vi "CallFacialClassificationFunction_IMA_DEPRECATEDQ.vi"(8 "error in (no error)":errorcluster, 9 "Function or Method Name":string="find_faces", 10 "image":T1, 11 "reference in":refnum<class "ImageFacialDetection.lvclass">) -> (0 "error out":errorcluster, 2 "image with faces":T1, 3 "reference out":refnum<class "ImageFacialDetection.lvclass">)   [LabVIEW 2017]
doc: "uses the image classification in python with openCV to detect faces in an image using Haar Cascades"
uses:
  ImageFacialDetection.lvclass
  <vilib>/Enthought/Python Integration Toolkit/Python Integration Toolkit.lvlib
  <vilib>/Enthought/Python Integration Toolkit/api/Unpack As Variant.vi
  <vilib>/vision/Image Controls.llb/IMAQ Image.ctl
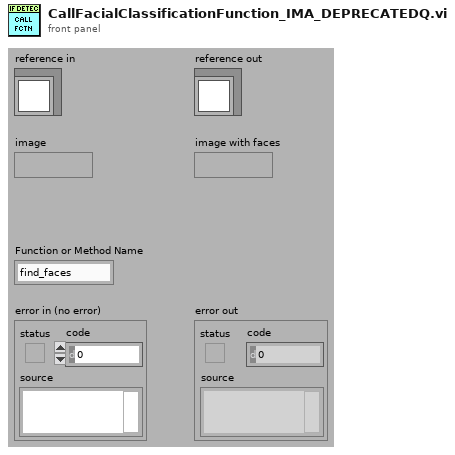
[diagram p1: front panel]
types:
  T1 = typedef "IMAQ Image.ctl" = refnum<image>
  T2 = typedef "Python Integration Toolkit.lvlib/Session ID.ctl" = u64
  T3 = typedef "Python Integration Toolkit.lvlib/Python Objects.ctl" = variant
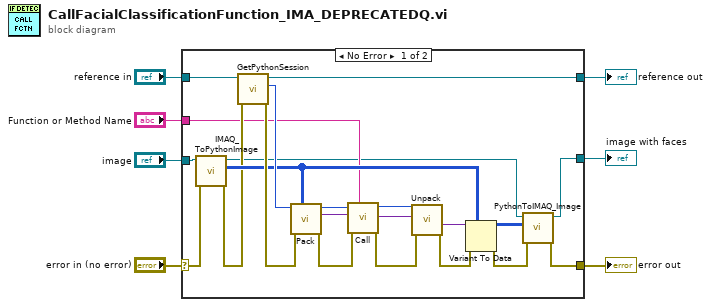
[diagram p0: block diagram]
diagram:
  n1 = case shown="No Error" "error in (no error)" {
    selector: "error in (no error)" -> [w18 w31]
    tunnel: [w11 w31] -> w6
    tunnel: [w28 w30] -> w4
    tunnel: "reference in" -> [w29 w30]
    tunnel: "image" -> [w27 _]
    tunnel: [w13 _] -> w2
    tunnel: "Function or Method Name" -> [w9 _]
    frame No Error {
      n2 = call "IMAQ_ToPythonImage.vi"("error in (no error)"=w18, "IMAQ Image in"=w27) -> ("error out"=w17:errorcluster, "Python Image Data"=w19:u8[][][], "IMAQ Image dup"=w8:T1)  [unwired: 7 in]
      n3 = call "GetPythonSession.vi"("error in (no error)"=w17, "reference in"=w29) -> ("error out"=w25:errorcluster, "Python Session ID"=w26:T2, "reference out"=w28:refnum<class "ImageFacialDetection.lvclass">)  [unwired: 7 in]
      n4 = call <vilib>:"Pack.vi"("Argument"=w19, "error in (no error)"=w25, "Session ID"=w26) -> ("error out"=w22:errorcluster, "Python Object References Out"=w23:T3, "Session ID out"=w24:T2)  [unwired: 6 in]
      n5 = call <vilib>:"Call.vi"("Function or Method Name"=w9, "error in (no error)"=w22, "Python Object References In"=w23, "Session ID"=w24) -> ("error out"=w15:errorcluster, "Python Object References Out"=w20:T3, "Session ID out"=w21:T2)  [unwired: 5 in]
      n6 = call-poly <vilib>:"Unpack.vi"("error in (no error)"=w15, "Python Object References In"=w20, "Session ID"=w21) -> ("error out"=w14:errorcluster, "Value"=w10:variant)  [unwired: 5 in, 2 out]
      n7 = Variant To Data(error in=w14, type=w19, Variant=w10) -> (data=w16:u8[][][], error out=w12:errorcluster)
      n8 = call "PythonToIMAQ_Image.vi"("error in (no error)"=w12, "Python Image"=w16, "IMAQ Image in"=w8) -> ("error out"=w11:errorcluster, "IMAQ Image out"=w13:T1)  [unwired: 7 in]
    }
    frame Error {
    }
  }
  "error out" <- w6
  "reference out" <- w4
  "image with faces" <- w2
